vi "PicoScopeospaGetStreamingLatestValues.vi"(0 "handle in":i16=16384, 1 "Polling Delays ms":T1={"Polling holdoff ms"=10, "Polling time ms"=90}, 2 "Buffer and Transfer Settings":T6={"startIndex"=0, "Samples"=1000000, "Down Sample Ratio"=1, "Down-Sample Mode"=2147483648} {"Down-Sample Mode" items=["RAW none"=2147483648, "None"=0, "Aggregate"=1, "Decimate"=2, "Average"=4]; "Down Sample Ratio" step=1; "Samples" format="%_6p"}, 3 "enabled array":i16[](array[numeric])=[1, 1, 0, 0, 0, 0, 0, 0, 0, 0], 5 "Device Info":T3, 7 "Data Pointers In":T4={"Max Buffer Pointers"=[], "Min Buffer Pointers"=[], "StreamingDataInfo"=[[{"Channel"=0, "Down-Sample Mode"=0, "PICO_DATA_TYPE"=enum."PICO_INT16_T", "Samples"=0, "bufferIndex"=0, "startIndex"=0, "overflow"=0}]]}, 9 "Buffer number":i32=1, 11 "error in (no error)":errorcluster) -> (4 "handle out":i16=16384, 8 "Data Pointers Out":T4={"Max Buffer Pointers"=[], "Min Buffer Pointers"=[], "StreamingDataInfo"=[[{"Channel"=0, "Down-Sample Mode"=0, "PICO_DATA_TYPE"=enum."PICO_INT16_T", "Samples"=0, "bufferIndex"=0, "startIndex"=0, "overflow"=0}]]}, 14 "tPicoStreamingDataTriggerInfo":T2, 15 "error out":errorcluster)   [LabVIEW 2010]
doc: "Call GetValues to fill a single set of channel buffers."
uses:
  psospa.dll
  shared/PicoBuffers.ctl
  shared/Buffer and Transfer Settings.ctl
panel:
  out "No of channels":u64=2
  in  "tPicoStreamingDataInfo":T5={"Channel"=0, "Down-Sample Mode"=2147483648, "PICO_DATA_TYPE"=enum."PICO_INT16_T", "Samples"=0, "bufferIndex"=0, "startIndex"=0, "overflow"=0} {"overflow" step=1 format="%010b"; "Down-Sample Mode" items=["None"=2147483648, "Aggregate"=1, "Decimate"=2, "Average"=4]; "Channel" items=["Channel A"=0, "Channel B"=1, "Channel C"=2, "Channel D"=3, "Channel E"=4, "Channel F"=5, "Channel G"=6, "Channel H"=7, "Port 0"=128, "Port 1"=129, "Trigger AUX"=1001]; "startIndex" step=1}
  in  "Streaming Acquisition Settings":T7={"preTriggerSamples"=0, "postTriggerSamples"=1000000, "Requested sampleInterval"=1.0, "sampleIntervalTimeUnits"=3} {"sampleIntervalTimeUnits" items=["femtoseconds", "picoseconds", "nanoseconds", "microseconds", "millseconds", "seconds"]; "postTriggerSamples" format="%_6p"; "preTriggerSamples" format="%_6p"}
  # "Samples can be equal to or less\nTotal Pre and Post Trigger Samples"
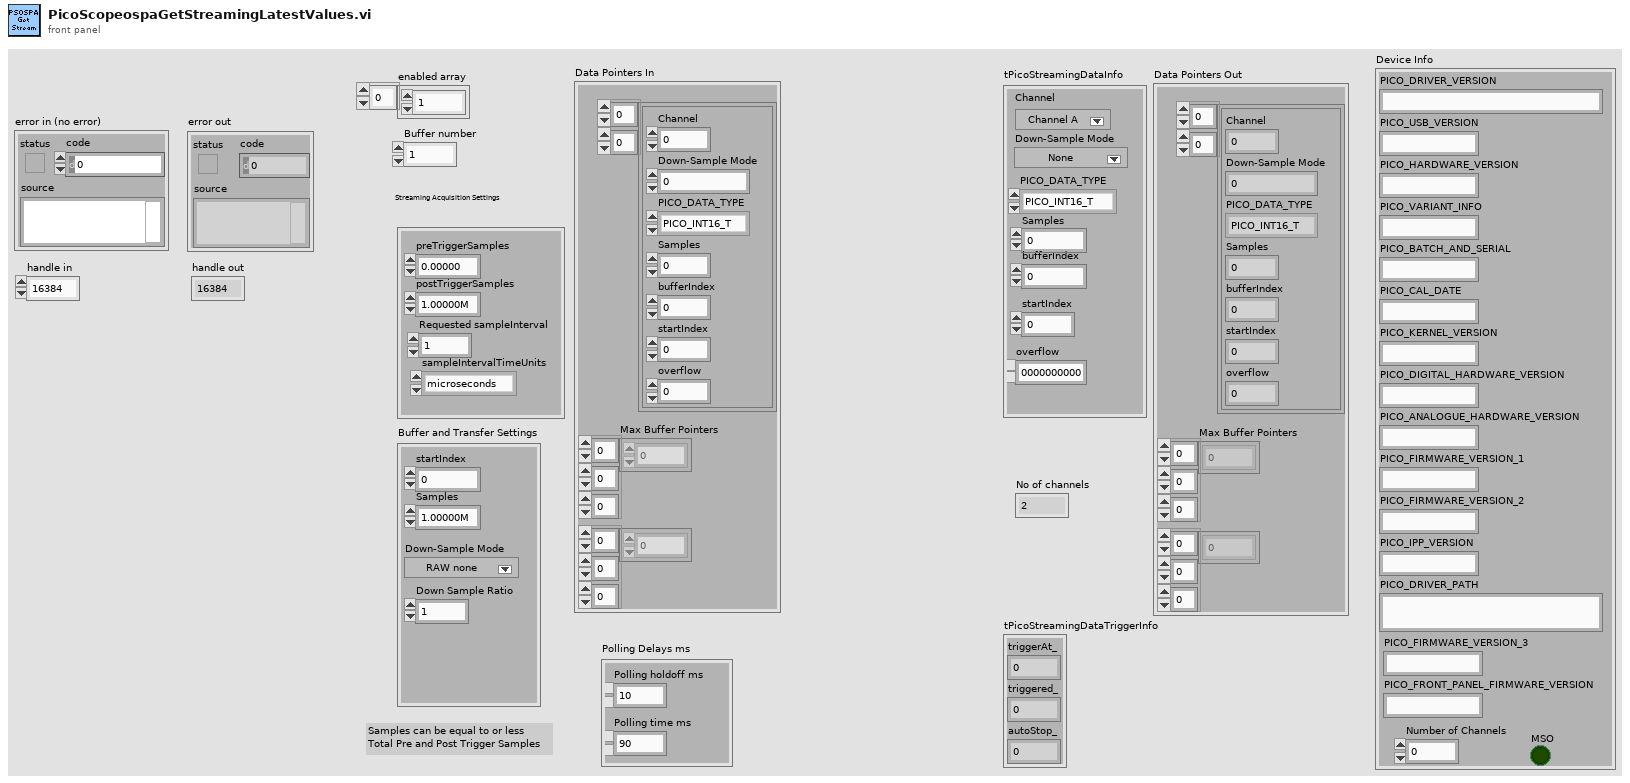
[diagram p1: front panel]
types:
  T1 = cluster{"Polling holdoff ms":u32, "Polling time ms":u32}
  T2 = cluster{"triggerAt_":u64, "triggered_":i16, "autoStop_":i16}
  T3 = cluster{"PICO_DRIVER_VERSION":string, "PICO_USB_VERSION":string, "PICO_HARDWARE_VERSION":string, "PICO_VARIANT_INFO":string, "PICO_BATCH_AND_SERIAL":string, "PICO_CAL_DATE":string, "PICO_KERNEL_VERSION":string, "PICO_DIGITAL_HARDWARE_VERSION":string, "PICO_ANALOGUE_HARDWARE_VERSION":string, "PICO_FIRMWARE_VERSION_1":string, "PICO_FIRMWARE_VERSION_2":string, "PICO_IPP_VERSION":string, "PICO_DRIVER_PATH":string, "PICO_FIRMWARE_VERSION_3":string, "PICO_FRONT_PANEL_FIRMWARE_VERSION":string, "Number of Channels":i16, "MSO":bool}
  T4 = typedef "PicoBuffers.ctl" = cluster{"Max Buffer Pointers":u64[][][], "Min Buffer Pointers":u64[][][], "StreamingDataInfo":cluster{"Channel":u32, "Down-Sample Mode":u32, "PICO_DATA_TYPE":enum32{"PICO_INT8_T", "PICO_INT16_T", "PICO_INT32_T", "PICO_UINT32_T", "PICO_INT64_T", ""}, "Samples":i32, "bufferIndex":u64, "startIndex":i32, "overflow":i16}[][]}
  T5 = cluster{"Channel":u32, "Down-Sample Mode":u32, "PICO_DATA_TYPE":enum32{"PICO_INT8_T", "PICO_INT16_T", "PICO_INT32_T", "PICO_UINT32_T", "PICO_INT64_T", ""}, "Samples":i32, "bufferIndex":u64, "startIndex":i32, "overflow":i16}
  T6 = typedef "Buffer and Transfer Settings.ctl" = cluster{"startIndex":u64, "Samples":u64, "Down Sample Ratio":u64, "Down-Sample Mode":u32}
  T7 = cluster{"preTriggerSamples":u64, "postTriggerSamples":u64, "Requested sampleInterval":dbl, "sampleIntervalTimeUnits":u32}
  T8 = cluster{"Channel":u32, "Down-Sample Mode":u32, "PICO_DATA_TYPE":enum32{"PICO_INT8_T", "PICO_INT16_T", "PICO_INT32_T", "PICO_UINT32_T", "PICO_INT64_T", ""}, "Samples":i32, "bufferIndex":u64, "startIndex":i32, "overflow":i16}[]
  T9 = cluster{"Channel":u32, "Down-Sample Mode":u32, "PICO_DATA_TYPE":enum32{"PICO_INT8_T", "PICO_INT16_T", "PICO_INT32_T", "PICO_UINT32_T", "PICO_INT64_T", ""}, "Samples":i32, "bufferIndex":u64, "startIndex":i32, "overflow":i16}[][]
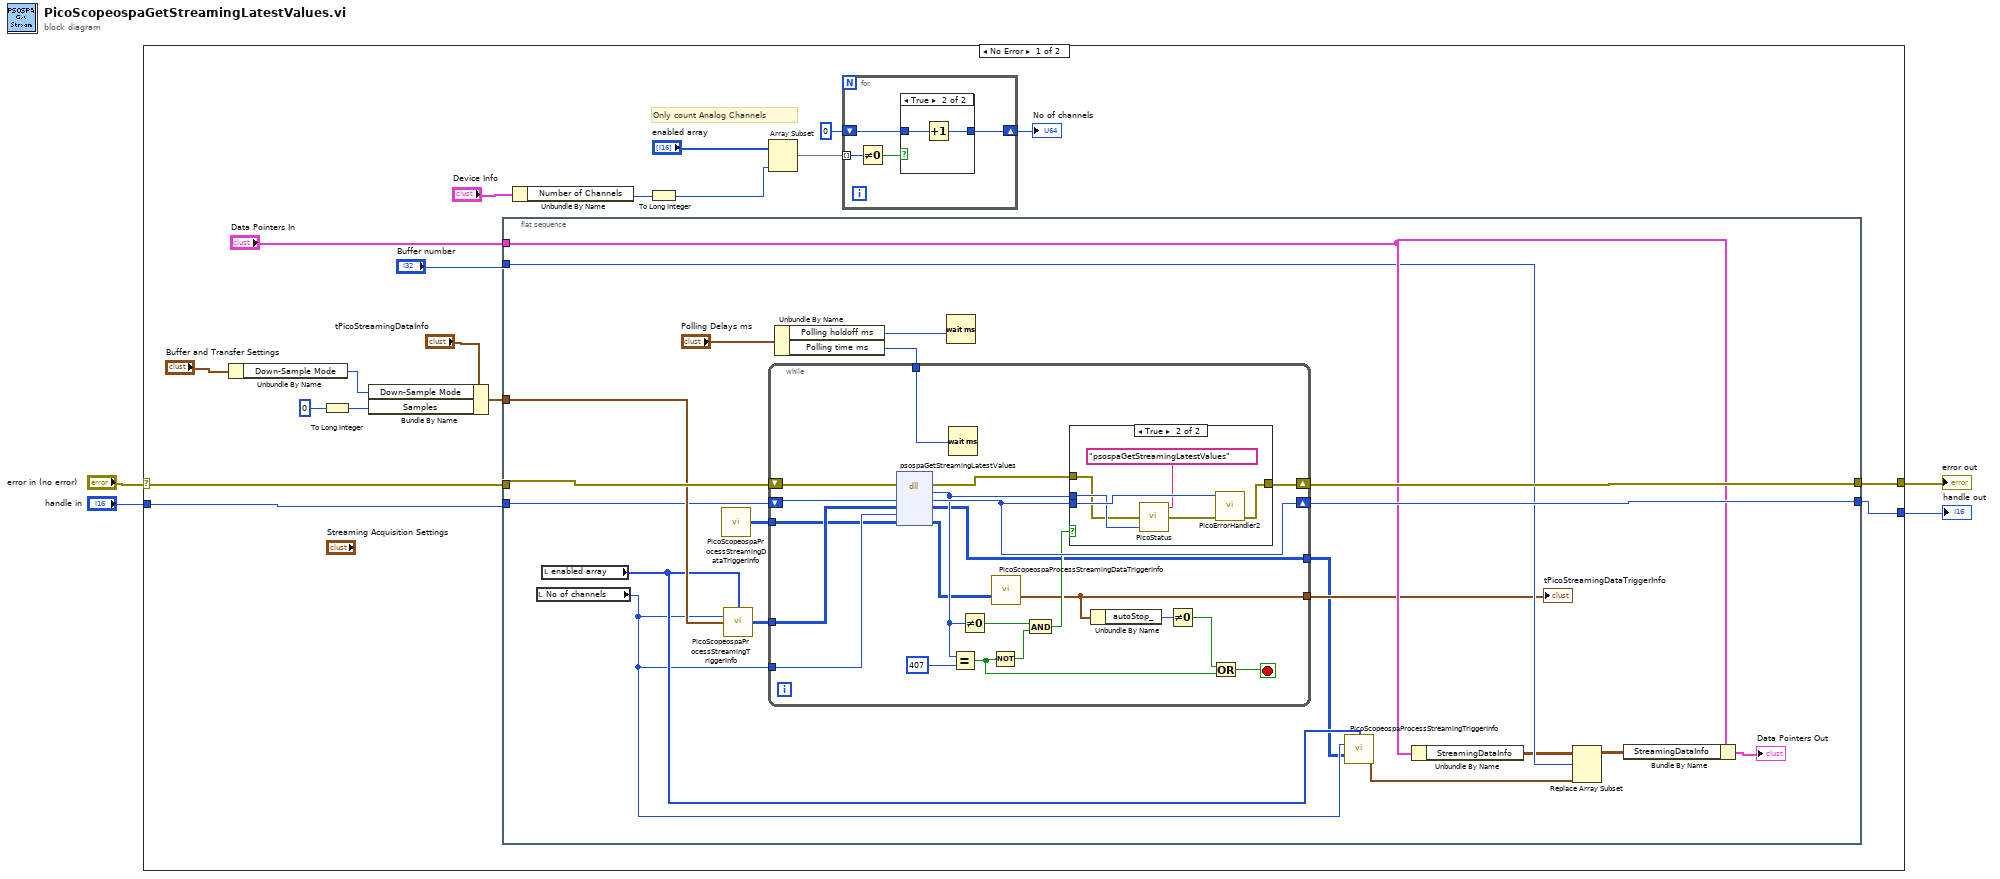
[diagram p0: block diagram]
diagram:
  n1 = case shown="No Error" "error in (no error)" {
    selector: "error in (no error)" -> [w20 w79]
    tunnel: "handle in" -> [w19 w80]
    tunnel: [w23 w80] -> w2
    tunnel: [w21 w79] -> w1
    frame No Error {
      # "Only count Analog Channels"
      n2 = Unbundle By Name("Buffer and Transfer Settings") -> ("Down-Sample Mode"=w15:u32)
      n3 = To Long Integer(number=0) -> (32bit integer=w14:i32)
      n4 = Bundle By Name(cluster="tPicoStreamingDataInfo", "Down-Sample Mode"=w15, "Samples"=w14) -> (w16:T5)
      n5 = flat-sequence {
        tunnel: w20 -> [w50]
        tunnel: w19 -> [w47]
        tunnel: "Buffer number" -> [w40]
        tunnel: w16 -> [w48]
        tunnel: [w46] -> w23
        tunnel: [w49] -> w21
        tunnel: "Data Pointers In" -> [w42]
        frame #0 {
          n6 = local read "No of channels"() -> (w36:u64)
          n7 = local read "enabled array"() -> (w37:i16[])
          n8 = call "PicoScopeospaProcessStreamingDataTriggerInfo.vi"() -> ("C Array for Struture Data Out"=w44:u16[][])  [unwired: 13 in, 2 out]
          n9 = call "PicoScopeospaProcessStreamingTriggerInfo.vi"("enabled array"=w37, "No of C Strutures"=w36, "C Struture define"=w48) -> ("C Array for Struture Data Out"=w43:u16[][])  [unwired: 10 in, 2 out]
          n10 = Unbundle By Name("Polling Delays ms") -> ("Polling holdoff ms"=w32:u32, "Polling time ms"=w31:u32)
          n11 = while {
            shift-right: [w69] -> w49
            shift-left: w50 -> [w71]
            shift-right: [w67] -> w46
            shift-left: w47 -> [w70]
            tunnel: w36 -> [w66]
            tunnel: w43 -> [w65]
            tunnel: w44 -> [w54]
            tunnel: [w58] -> w38
            tunnel: w31 -> [w52]
            tunnel: [w51] -> w35
            stop <- w53 stop-if-true
            n12 = dll-call lib="psospa.dll" fn="psospaGetStreamingLatestValues" ("ps3000.dll:_ps3000_open_unit@0")(error in=w71, "handle"=w70, "streamingDataInfo"=w65, "nStreamingDataInfos"=w66, "triggerInfo"=w54) -> (error out=w68:errorcluster, "PICO_STATUS"=w63:u32, "handle"=w67:i16, "streamingDataInfo"=w51:u16[][], "triggerInfo"=w59:u16[][])  [unwired: 3 in, 1 out]
            n13 = Wait (ms)(milliseconds to wait=w52) -> ()  [unwired: 1 out]
            n14 = Equal?(x=w63, y=u32 407) -> (x = y?=w56:bool)
            n15 = Not Equal To 0?(x=w63) -> (x != 0?=w61:bool)
            n16 = Not(x=w56) -> (.not. x?=w60:bool)
            n17 = call "PicoScopeospaProcessStreamingDataTriggerInfo.vi"("C Array for Struture Data In"=w59) -> ("tPicoStreamingDataTriggerInfo"=w58:T2)  [unwired: 12 in, 2 out]
            n18 = And(x=w61, y=w60) -> (x .and. y?=w62:bool)
            n19 = case shown="True" w62 {
              tunnel: w67 -> [_ w78]
              tunnel: [w72 w77] -> w69
              tunnel: w63 -> [_ w76]
              tunnel: w68 -> [w72 w75]
              frame False {
              }
              frame True {
                n20 = call "PicoStatus.vi"("PICO STATUS"=w76, "error in"=w75, "source"="psospaGetStreamingLatestValues") -> ("error out"=w73:errorcluster)
                n21 = call "PicoErrorHandler2.vi"("error in (no error)"=w73, "handle In"=w78) -> ("error out"=w77:errorcluster)  [unwired: 9 in]
              }
            }
            n22 = Unbundle By Name(w58) -> ("autoStop_"=w57:i16)
            n23 = Not Equal To 0?(x=w57) -> (x != 0?=w55:bool)
            n24 = Or(x=w55, y=w56) -> (x .or. y?=w53:bool)
          }
          "tPicoStreamingDataTriggerInfo" <- w38
          n25 = Wait (ms)(milliseconds to wait=w32) -> ()  [unwired: 1 out]
          n26 = call "PicoScopeospaProcessStreamingTriggerInfo.vi"("enabled array"=w37, "No of C Strutures"=w36, "C Array for Struture Data In"=w35) -> ("Array of Clusters"=w34:T8)  [unwired: 10 in, 2 out]
          n27 = Unbundle By Name(w42) -> ("StreamingDataInfo"=w39:T9)
          n28 = Replace Array Subset(array=w39, new element=w34, index (row)=w40) -> (w41:T9)  [unwired: 1 in]
          n29 = Bundle By Name(cluster=w42, "StreamingDataInfo"=w41) -> (→"Data Pointers Out":T4)
        }
      }
      n30 = Unbundle By Name("Device Info") -> ("Number of Channels"=w11:i16)
      n31 = To Long Integer(number=w11) -> (32bit integer=w9:i32)
      n32 = Array Subset(array="enabled array", length=w9) -> (w5:i16[])  [unwired: 1 in]
      n33 = for {
        shift-right: [w27] -> w8
        shift-left: u64 0 -> [w26]
        tunnel: w5 -> [w25] mode=indexing
        n34 = Not Equal To 0?(x=w25) -> (x != 0?=w24:bool)
        n35 = case shown="True" w24 {
          tunnel: [w28 w30] -> w27
          tunnel: w26 -> [w28 w29]
          frame False {
          }
          frame True {
            n36 = Increment(x=w29) -> (x+1=w30:u64)
          }
        }
      }
      "No of channels" <- w8
    }
    frame Error {
    }
  }
  "handle out" <- w2
  "error out" <- w1
